vi "ECG-WAVELET.vi"() -> ()   [LabVIEW 2018]
panel:
  out "ECG":dynamicdata(graph)
  out "ECG-WAVELET":waveform(dbl)(graph)
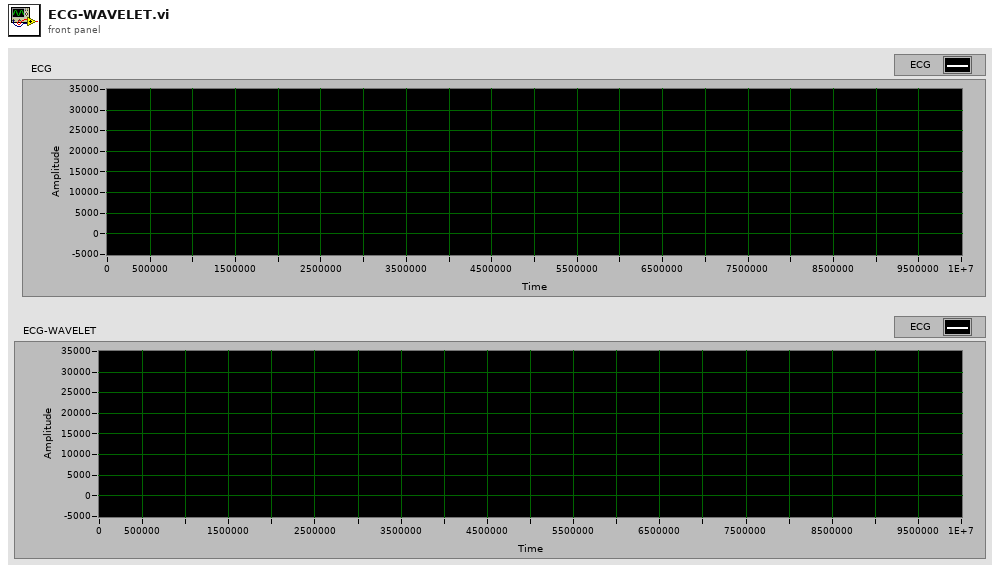
[diagram p1: front panel]
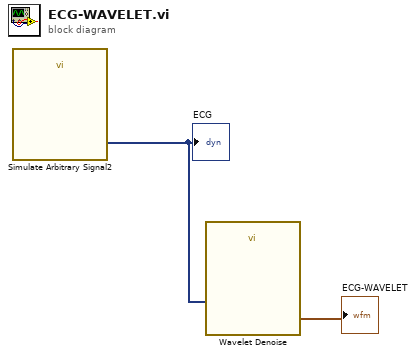
[diagram p0: block diagram]
diagram:
  n1 = call "Simulate Arbitrary Signal2"() -> ("Signal"=w1:dynamicdata)  [unwired: 9 in, 2 out]
  "ECG" <- w1
  n2 = call "Wavelet Denoise"("Signal"=w1) -> ("Denoised Signal"=→"ECG-WAVELET":waveform(dbl))  [unwired: 9 in, 1 out]
